vi "REV RPM to ft per s.vi"() -> ()   [LabVIEW 2020]
panel:
  in  "RPM":dbl
  out "ft/s":dbl
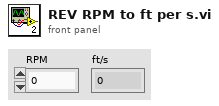
[diagram p1: front panel]
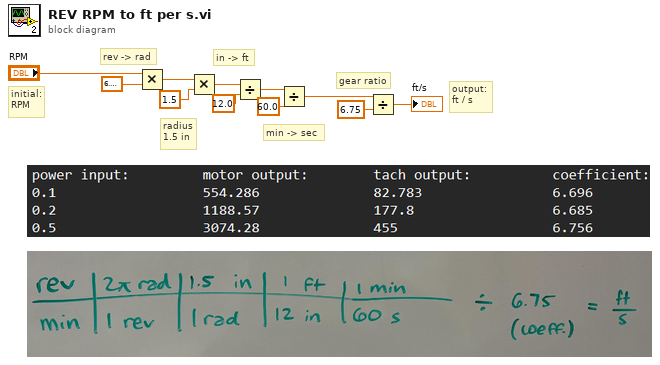
[diagram p0: block diagram]
diagram:
  # "output:\nft / s"
  # "gear ratio"
  # "min -> sec"
  # "in -> ft"
  # "initial:\nRPM"
  # "radius\n1.5 in"
  # "rev -> rad"
  n1 = Multiply(x="RPM", y=6.283185307179586) -> (x*y=w10:dbl)
  n2 = Multiply(x=w10, y=1.5) -> (x*y=w8:dbl)
  n3 = Divide(x=w8, y=12.0) -> (x/y=w6:dbl)
  n4 = Divide(x=w6, y=60.0) -> (x/y=w4:dbl)
  n5 = Divide(x=w4, y=6.75) -> (x/y=→"ft/s":dbl)
